vi "Cleanup.vi"(8 "error in (no error)":errorcluster, 11 "Concrete Message Rescripter in":refnum<class "Concrete Message Rescripter.lvclass">) -> (0 "error out":errorcluster, 3 "Concrete Message Rescripter out":refnum<class "Concrete Message Rescripter.lvclass">)   [LabVIEW 2020, in "Message Rescripter.lvlib" / "Concrete Message Rescripter.lvclass"]
uses:
  Concrete Message Rescripter.lvclass
  MessageMakerProvider/_Message Maker/_Maker Classes/Concrete Message Scripter/Concrete Message Scripter.lvclass
  Message Rescripter.lvlib
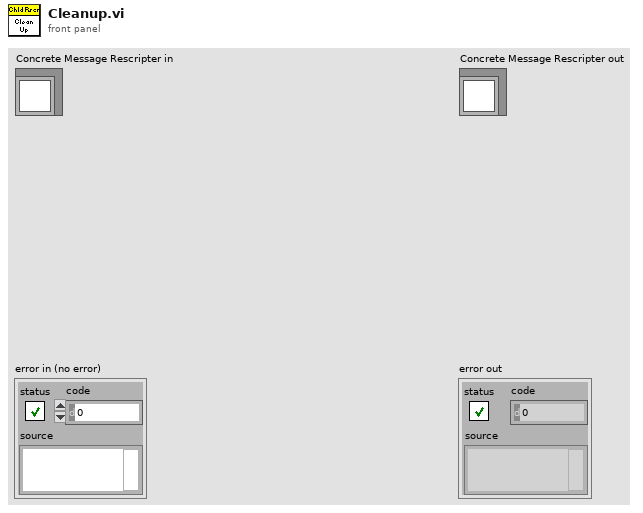
[diagram p1: front panel]
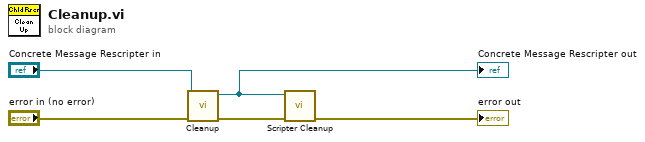
[diagram p0: block diagram]
diagram:
  n1 = call-parent "Cleanup.vi"("error in (no error)"="error in (no error)", "Message Scripter in"="Concrete Message Rescripter in") -> ("error out"=w4:errorcluster, "Message Scripter out"=w2:refnum<class "Concrete Message Rescripter.lvclass">)  [unwired: 8 in]
  "Concrete Message Rescripter out" <- w2
  n2 = call "Scripter Cleanup.vi"("error in (no error)"=w4, "Coupled Message Rescripter in"=w2) -> ("error out"=→"error out":errorcluster)  [unwired: 9 in]
